vi "PBx Run.vi"(8 "error in":errorcluster, 11 "RT Data In":T1) -> (0 "error out":errorcluster, 3 "RT Data Out":T1)   [LabVIEW 2015]
uses:
  DCM-NIVS-RT/Compiled Data.ctl
  Types/RT Data.ctl
  DCM Engine.lvlib
  <vilib>/NI VeriStand/Custom Device Waveform API/Multiple Waveforms Write (DBL)/Multiple Waveforms Write (DBL).lvclass
  <vilib>/NI Veristand/Custom Device API/Waveform Data Reference.ctl
  <vilib>/NI VeriStand/Custom Device API/Custom Device API.lvlib
  DCM-NIVS-RT/PB-01.ctl
  <vilib>/Powertrain Controls/Device Drivers/Engine Position Tracking/EPTx/RevA/RT/Controls/EPTxFilters.ctl
  <vilib>/Powertrain Controls/Device Drivers/Engine Position Tracking/EPTx/RevA/RT/EPTx - RevA - RT.lvlib
  <vilib>/Powertrain Controls/Device Drivers/DCM/Rev0/RT/Configuration.ctl
  <vilib>/Powertrain Controls/Device Drivers/DCM/Rev0/RT/DCM - RT.lvclass
  <vilib>/Powertrain Controls/Device Drivers/DCM/Rev0/RT/System Settings.ctl
  <vilib>/Powertrain Controls/Device Drivers/DCM/DI/RT/Phase.ctl
  <vilib>/Powertrain Controls/Device Drivers/DCM/DI/RT/DCM - RT - DI.lvlib
  <vilib>/Powertrain Controls/Device Drivers/DCM/Rev0/FPGA/Digital Channel.ctl
  <vilib>/Powertrain Controls/Device Drivers/DCM/Rev0/FPGA/DCM - FPGA.lvlib
  <vilib>/Powertrain Controls/Device Drivers/DCM/Rev0/FPGA/DI - Bank Configuration.ctl
  <vilib>/Powertrain Controls/Device Drivers/DCM/Rev0/RT/User LED.ctl
  <vilib>/Powertrain Controls/Device Drivers/DCM/HH/RT/Duration Pre Scale.ctl
  <vilib>/Powertrain Controls/Device Drivers/DCM/HH/RT/DCM - RT - HH.lvlib
  <vilib>/Powertrain Controls/Device Drivers/DCM/Rev0/FPGA/DI - Drive State.ctl
  <vilib>/Powertrain Controls/Device Drivers/DCM/DI/FPGA/Phase Step.ctl
  <vilib>/Powertrain Controls/Device Drivers/DCM/DI/FPGA/DCM - FPGA - DI.lvlib
  <vilib>/Powertrain Controls/Device Drivers/DCM/DI/FPGA/Control.ctl
  <vilib>/Powertrain Controls/Device Drivers/VR-Hall/RevC/Real-Time/Support/Vr_Hall_mode_control_revc.ctl
  DCM-NIVS-RT/Engine Init Data.ctl
  DCM-NIVS-RT/Engine Status.ctl
  DCM-NIVS-RT/EPTx Signal Select.ctl
  DCM-NIVS-RT/EPTx RevA RT Data.ctl
  DCM-NIVS-RT/DiffIO Results Indexes.ctl
  DCM-NIVS-RT/DiffIO Setup Indexes.ctl
  DCM-NIVS-RT/DiffIO.ctl
  DCM-NIVS-RT/HH Command Indexes.ctl
  DCM-NIVS-RT/HH.ctl
  DCM-NIVS-RT/DI Scope.ctl
  DCM-NIVS-RT/User OS.ctl
  DCM-NIVS-RT/HH Config Indexes.ctl
  DCM-NIVS-RT/HH Status Indexes.ctl
  DCM-NIVS-RT/DI Faults Indexes.ctl
  DCM-NIVS-RT/System State Indexes.ctl
  DCM-NIVS-RT/DCM Core.ctl
  DCM-NIVS-RT/ESTTL Setup Indexes.ctl
  DCM-NIVS-RT/PBx.ctl
  DCM-NIVS-RT/Knock.ctl
  DCM-NIVS-RT/HH Scope.ctl
  DCM-NIVS-RT/DI Command Indexes.ctl
  DCM-NIVS-RT/DI Phase Outputs.ctl
  DCM-NIVS-RT/DI.ctl
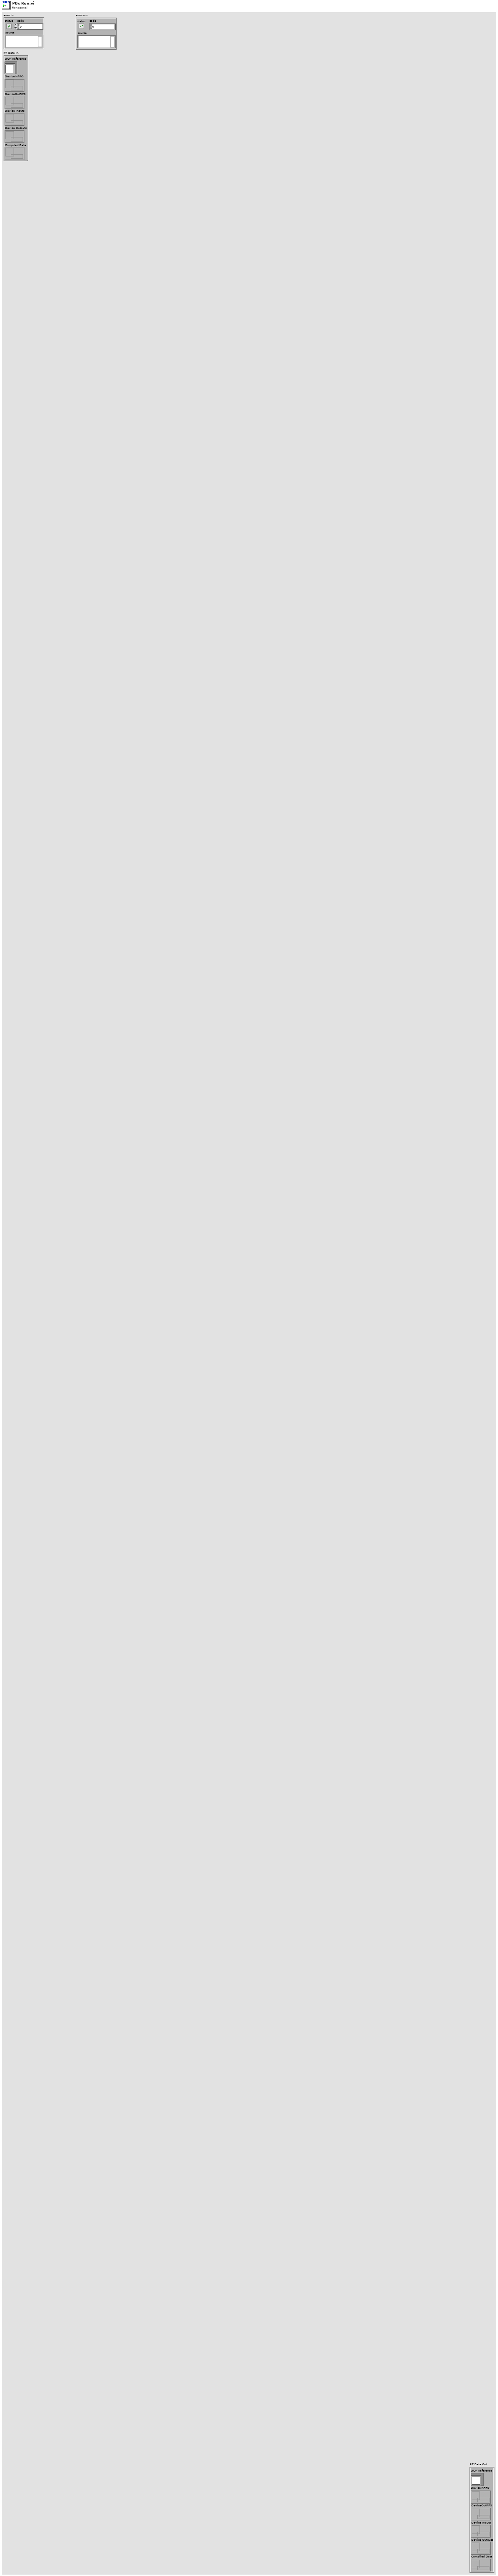
[diagram p1: front panel]
types:
  T1 = typedef "DCM Engine.lvlib/RT Data.ctl" = cluster{"DCM Reference":refnum<class "DCM - RT.lvclass">, "DeviceInFIFO":refnum<k33>, "DeviceOutFIFO":refnum<k33>, "Device Inputs":refnum<data-value>, "Device Outputs":refnum<data-value>, "Compiled Data":refnum<data-value>}
  T2 = typedef "DCM Shared.lvlib/PBx.ctl" = cluster{"PB Version":u8, "PB-01":T3}
  T3 = typedef "DCM Shared.lvlib/PB-01.ctl" = cluster{"FIFO Indexes":cluster{"Write":cluster{"Clear Faults":i32, "ESTTL Setup":T4[], "UEGO Control":cluster{"UEGO1Enable":i32, "UEGO2Enable":i32, "UEGO1Range":i32, "UEGO2Range":i32, "FilterCutoff (Hz)":i32}}, "Read":cluster{"UEGO Sensor Results":cluster{"UEGO1Lambda":i32, "UEGO1Phi":i32, "UEGO1AFRatio":i32, "UEGO1Ip (mA)":i32, "UEGO2Lambda":i32, "UEGO2Phi":i32, "UEGO2AFRatio":i32, "UEGO2Ip (mA)":i32}, "UEGO Temperature (C)":cluster{"UEGO1Temp (C)":i32, "UEGO2Temp (C)":i32, "UEGO1Hot":i32, "UEGO2Hot":i32}, "UEGO Diagnostics":cluster{"UEGO1SensorFault":i32, "UEGO2SensorFault":i32, "UEGO1HeaterFault":i32, "UEGO2HeaterFault":i32, "UEGOFuseStatus":i32, "Battery (V)":i32, "LSUType":i32}}}, "Settings":cluster{"VR-Hall Mode Select":T5[], "VR-Hall Arming Threshold [V]":dbl[], "ESTTL Command Enabled":bool}}
  T4 = typedef "ESTTL Setup Indexes.ctl" = cluster{"Mode":i32, "Polarity":i32, "Frequency [Hz]":i32, "Duty Cycle [%]":i32, "TDC Offset [CAD]":i32, "Window Start [DBTDC]":i32, "Window End [DBTDC]":i32, "Angles":cluster{"Enable":i32, "Location [DBTDC]":i32, "Duration [s]":i32}[], "Skip Fire":i32, "Skip Fire Index":i32}
  T5 = typedef "Vr_Hall_mode_control_revc.ctl" = enum32{"VR Adaptive Arm", "VR Manual Arm", "Hall", "Hall w/ Pull-up"}
  T6 = typedef "PB-01.ctl" = cluster{"FIFO Indexes":cluster{"Write":cluster{"Clear Faults":i32, "ESTTL Setup":T4[], "UEGO Control":cluster{"UEGO1Enable":i32, "UEGO2Enable":i32, "UEGO1Range":i32, "UEGO2Range":i32, "FilterCutoff (Hz)":i32}}, "Read":cluster{"UEGO Sensor Results":cluster{"UEGO1Lambda":i32, "UEGO1Phi":i32, "UEGO1AFRatio":i32, "UEGO1Ip (mA)":i32, "UEGO2Lambda":i32, "UEGO2Phi":i32, "UEGO2AFRatio":i32, "UEGO2Ip (mA)":i32}, "UEGO Temperature (C)":cluster{"UEGO1Temp (C)":i32, "UEGO2Temp (C)":i32, "UEGO1Hot":i32, "UEGO2Hot":i32}, "UEGO Diagnostics":cluster{"UEGO1SensorFault":i32, "UEGO2SensorFault":i32, "UEGO1HeaterFault":i32, "UEGO2HeaterFault":i32, "UEGOFuseStatus":i32, "Battery (V)":i32, "LSUType":i32}}}, "Settings":cluster{"VR-Hall Mode Select":T5[], "VR-Hall Arming Threshold [V]":dbl[], "ESTTL Command Enabled":bool}}
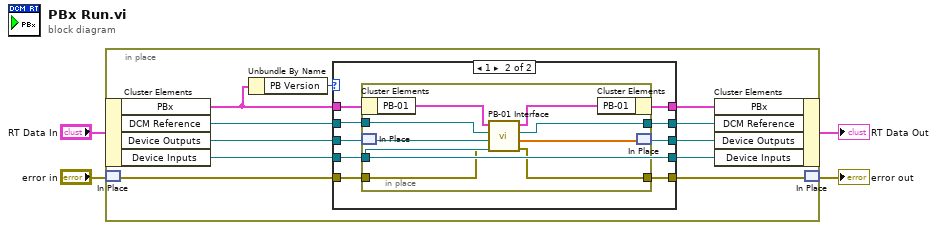
[diagram p0: block diagram]
diagram:
  n1 = in-place {
    n2 = in-place-cluster #1("RT Data In") -> ("PBx"=w14:T2, "DCM Reference"=w13:refnum<class "DCM - RT.lvclass">, "Device Outputs"=w12:refnum<data-value>, "Device Inputs"=w11:refnum<data-value>)
    n3 = in-place-match #2("error in") -> (w6:errorcluster)
    n4 = Unbundle By Name(w14) -> ("PB Version"=w15:u8)
    n5 = case shown="1" w15 {
      tunnel: w14 -> [w20 w29]
      tunnel: w13 -> [w19 w22]
      tunnel: w12 -> [w18 w28]
      tunnel: w11 -> [w17 w27]
      tunnel: [w20 w25] -> w10
      tunnel: [w19 w21] -> w9
      tunnel: [w18 w26] -> w8
      tunnel: [w17 w27] -> w7
      tunnel: [w16 w23] -> w5
      tunnel: w6 -> [w16 w24]
      frame 0, Default {
      }
      frame 1 {
        n6 = in-place {
          in-place-border: w27 -> [w35]
          in-place-border: w24 -> [w33]
          in-place-border: [w32] -> w23
          in-place-border: w22 -> [w31]
          in-place-border: [w30] -> w21
          n7 = in-place-cluster #3(w29) -> ("PB-01"=w38:T3)
          n8 = in-place-match #4(w28) -> (w36:refnum<data-value>)
          n9 = call "PB-01 Interface.vi"("Device Inputs"=w35, "error in"=w33, "Device Outputs in"=w36, "DCM Ref"=w31, "PB-01 in"=w38) -> ("error out"=w32:errorcluster, "Device Outputs out"=w34:dbl[], "DCM Ref"=w30:refnum<class "DCM - RT.lvclass">, "PB-01 out"=w37:T6)  [unwired: 3 in]
          n10 = in-place-cluster #3("PB-01"=w37) -> (w25:T2)
          n11 = in-place-match #4(w34) -> (w26:refnum<data-value>)
        }
      }
    }
    n12 = in-place-cluster #1("PBx"=w10, "DCM Reference"=w9, "Device Outputs"=w8, "Device Inputs"=w7) -> (→"RT Data Out":T1)
    n13 = in-place-match #2(w5) -> (→"error out":errorcluster)
  }
